vi "Begin.vi"(8 "error in":errorcluster) -> (0 "error out":errorcluster)   [LabVIEW 2017]
doc: "Called before other user functions, this VI is expected to open initial I/O refnums, load in file data, and do all program initialization. Notice that the <B>error out</B> terminal is simply used for data flow. Wiring it to other structures or subVIs ensures that this VI runs first."
uses:
  <vilib>/Rock Robotics/SystemInterfaces/DIO/FPGA_DIOPWMChannel.ctl
  <vilib>/Rock Robotics/WPI/DriverStation/WPI_DriverStationRobotMode2.ctl
  <vilib>/Rock Robotics/WPI/Joystick/WPI_JoystickDeviceEnum.ctl
  <vilib>/Rock Robotics/WPI/SafetyOutput/WPI_SafetyOutputConfigMenu.ctl
  <vilib>/Rock Robotics/WPI/RobotDrive/WPI_RobotDriveOpen2MotorWithSPARK.vi
  Robot Global Data.vi
  <vilib>/Rock Robotics/Network Tables/NT Write String Array.vi
  <vilib>/Rock Robotics/WPI/MotorControl/WPI_MotorControlOpen SPARK.vi
  <vilib>/NI_Real-Time Target Support.lvlib
panel:
  out "Led State":bool
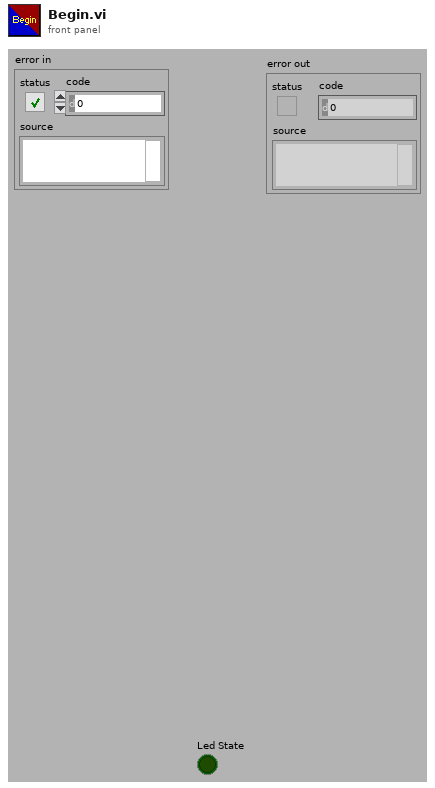
[diagram p1: front panel]
types:
  T1 = typedef "FPGA_DIOPWMChannel.ctl" = enum8{"PWM 0", "PWM 1", "PWM 2", "PWM 3", "PWM 4", "PWM 5", "PWM 6", "PWM 7", "PWM 8", "PWM 9", "PWM MXP 0", "PWM MXP 1", "PWM MXP 2", "PWM MXP 3", "PWM MXP 4", "PWM MXP 5", "PWM MXP 6", "PWM MXP 7", "PWM MXP 8", "PWM MXP 9", "Invalid"}
  T2 = typedef "WPI_SafetyOutputConfigMenu.ctl" = enum16{"Enable", "Disable"}
  T3 = typedef "WPI_JoystickDeviceEnum.ctl" = enum16{"USB 0", "USB 1", "USB 2", "USB 3", "USB 4", "USB 5"}
  T4 = typedef "WPI_DriverStationRobotMode2.ctl" = enum16{"Autonomous Disabled", "Autonomous Enabled", "Teleop Disabled", "Teleop Enabled", "Disconnected", "Finish", "Test Disabled", "Test Enabled", "Emergency Stopped"}
  T5 = typedef "WPI_JoystickDevRef.ctl" = cluster{"Device":T3}
  T6 = typedef "WPI_MotorControlDeviceRef.ctl" = cluster{"DeviceStatus":errorcluster, "Type":T7, "PWM":cluster{"PWM Channel":T1, "DeadBand":T8}, "CAN":cluster{"Device Number":u8, "SetOutput VI Ref":variant, "GetOutput VI Ref":variant, "Enable VI Ref":variant, "Disable VI Ref":variant, "Data":variant}, "Invert":bool, "DIO PWM":cluster{"PWM \"Enable\" Channel":T1, "DIOChannel":T9, "PWM Rate":dbl}}
  T7 = typedef "WPI_MotorControlType.ctl" = enum16{"PWM", "CAN", "DIO PWM"}
  T8 = typedef "WPI_PWMDeadband.ctl" = cluster{"Name":string, "maxPositivePwm":i32, "minPositivePwm":i32, "centerPwm":i32, "maxNegativePwm":i32, "minNegativePwm":i32, "angularRange":u16}
  T9 = typedef "FPGA_DIOChannel.ctl" = enum8{"DIO 0", "DIO 1", "DIO 2", "DIO 3", "DIO 4", "DIO 5", "DIO 6", "DIO 7", "DIO 8", "DIO 9", "DIO MXP 0", "DIO MXP 1", "DIO MXP 2", "DIO MXP 3", "DIO MXP 4", "DIO MXP 5", "DIO MXP 6", "DIO MXP 7", "DIO MXP 8", "DIO MXP 9", "DIO MXP 10", "DIO MXP 11", "DIO MXP 12", "DIO MXP 13", "DIO MXP 14", "DIO MXP 15", "SPI Port CS1", "SPI Port CS2", "SPI Port CS3", "SPI Port MISO", "SPI Port MOSI", "Invalid"}
  T10 = typedef "WPI_RobotDriveDevRef.ctl" = cluster{"DevStatus":errorcluster, "Motors[]":T6[], "Square Inputs":bool, "Max Output":dbl}
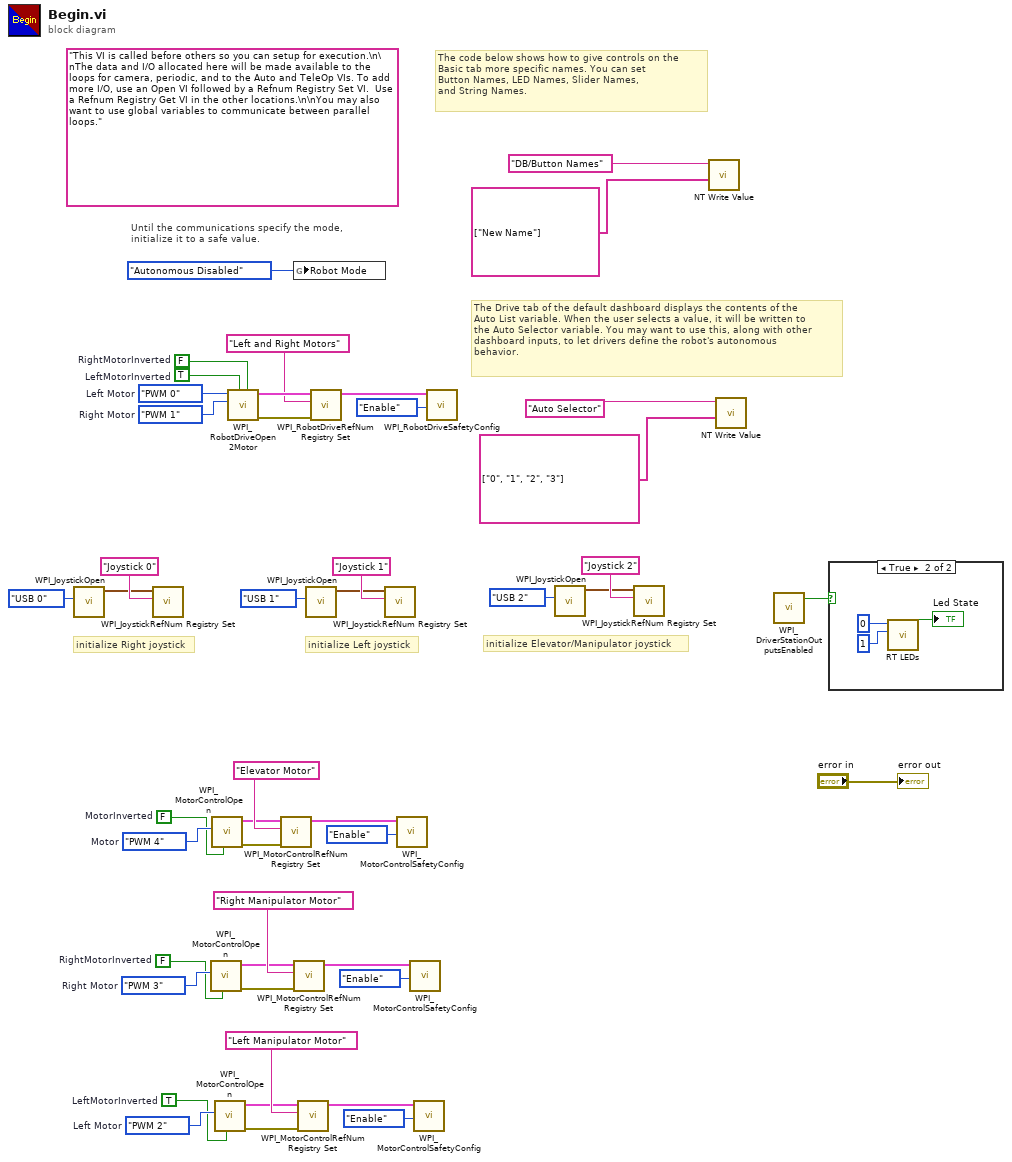
[diagram p0: block diagram]
diagram:
  w5 = FPGA_DIOPWMChannel."PWM 4"  # Motor
  w4 = FALSE  # MotorInverted
  w13 = FPGA_DIOPWMChannel."PWM 2"  # Left Motor
  w6 = TRUE  # LeftMotorInverted
  w24 = FPGA_DIOPWMChannel."PWM 3"  # Right Motor
  w7 = FALSE  # RightMotorInverted
  (unwired) "This VI is called before others so you can setup for execution.\n\nThe data and I/O allocated here will be made available to the loops for camera, periodic, and to the Auto and TeleOp VIs. To add more I/O, use an Open VI followed by a Refnum Registry Set VI.  Use a Refnum Registry Get VI in the other locations.\n\nYou may also want to use global variables to communicate between parallel loops."
  w40 = FPGA_DIOPWMChannel."PWM 1"  # Right Motor
  w41 = FPGA_DIOPWMChannel."PWM 0"  # Left Motor
  w45 = TRUE  # LeftMotorInverted
  w46 = FALSE  # RightMotorInverted
  # "initialize Elevator/Manipulator joystick"
  # "initialize Right joystick"
  # "The Drive tab of the default dashboard displays the contents of the\nAuto List variable. When the user selects a value, it will be written to\nthe Auto Selector variable. You may want to use this, along with other\ndashboard inputs, to let drivers define the robot's autonomous\nbehavior."
  # "The code below shows how to give controls on the\nBasic tab more specific names. You can set\nButton Names, LED Names, Slider Names,\nand String Names."
  # "initialize Left joystick"
  # "Until the communications specify the mode,\ninitialize it to a safe value."
  n1 = call <vilib>:"WPI_JoystickOpen.vi"("JoystickDevice"=WPI_JoystickDeviceEnum."USB 0") -> ("JoystickDevRef"=w21:T5)  [unwired: 10 in]
  n2 = call <vilib>:"WPI_JoystickRefNum Registry Set.vi"("refnum name"="Joystick 0", "JoystickDevRef"=w21) -> ()  [unwired: 8 in, 2 out]
  n3 = call-poly <vilib>:"WPI_MotorControlOpen.vi"("Invert"=w7, "PWM Channel"=w24) -> ("error out"=w25:errorcluster, "MotorControlDeviceRef"=w9:T6)  [unwired: 8 in]
  n4 = call-poly <vilib>:"WPI_MotorControlOpen.vi"("Invert"=w4, "PWM Channel"=w5) -> ("error out"=w3:errorcluster, "MotorControlDeviceRef"=w1:T6)  [unwired: 8 in]
  n5 = call-poly <vilib>:"WPI_MotorControlOpen.vi"("Invert"=w6, "PWM Channel"=w13) -> ("error out"=w14:errorcluster, "MotorControlDeviceRef"=w10:T6)  [unwired: 8 in]
  n6 = call-poly <vilib>:"WPI_RobotDriveOpen2Motor.vi"("Right Motor Inverted"=w46, "Left Motor Inverted"=w45, "Right Motor"=w40, "Left Motor"=w41) -> ("error out"=w42:errorcluster, "RobotDriveDevRef"=w44:T10)  [unwired: 6 in]
  n7 = call <vilib>:"WPI_MotorControlRefNum Registry Set.vi"("error in (no error)"=w3, "refnum name"="Elevator Motor", "MotorControlDevRef"=w1) -> ("MotorControlDevRef"=w16:T6)  [unwired: 7 in, 1 out]
  n8 = global write "Robot Global Data.vi" "Robot Mode"(WPI_DriverStationRobotMode2."Autonomous Disabled" ("Robot Mode")) -> ()
  n9 = call <vilib>:"WPI_MotorControlRefNum Registry Set.vi"("error in (no error)"=w25, "refnum name"="Right Manipulator Motor", "MotorControlDevRef"=w9) -> ("MotorControlDevRef"=w8:T6)  [unwired: 7 in, 1 out]
  n10 = call <vilib>:"WPI_MotorControlRefNum Registry Set.vi"("error in (no error)"=w14, "refnum name"="Left Manipulator Motor", "MotorControlDevRef"=w10) -> ("MotorControlDevRef"=w11:T6)  [unwired: 7 in, 1 out]
  n11 = call <vilib>:"WPI_JoystickOpen.vi"("JoystickDevice"=WPI_JoystickDeviceEnum."USB 1") -> ("JoystickDevRef"=w35:T5)  [unwired: 10 in]
  n12 = call <vilib>:"WPI_RobotDriveRefNum Registry Set.vi"("error in (no error)"=w42, "refnum name"="Left and Right Motors", "RobotDriveDevRef"=w44) -> ("RobotDriveDevRef"=w39:T10)  [unwired: 1 in, 7 out]
  n13 = call <vilib>:"WPI_JoystickRefNum Registry Set.vi"("refnum name"="Joystick 1", "JoystickDevRef"=w35) -> ()  [unwired: 8 in, 2 out]
  n14 = call <vilib>:"WPI_MotorControlSafetyConfig.vi"("mode"=WPI_SafetyOutputConfigMenu."Enable", "MotorControlDevRef"=w16) -> ()  [unwired: 8 in, 2 out]
  n15 = call <vilib>:"WPI_MotorControlSafetyConfig.vi"("mode"=WPI_SafetyOutputConfigMenu."Enable", "MotorControlDevRef"=w8) -> ()  [unwired: 8 in, 2 out]
  n16 = call <vilib>:"WPI_MotorControlSafetyConfig.vi"("mode"=WPI_SafetyOutputConfigMenu."Enable", "MotorControlDevRef"=w11) -> ()  [unwired: 8 in, 2 out]
  n17 = call <vilib>:"WPI_RobotDriveSafetyConfig.vi"("mode"=WPI_SafetyOutputConfigMenu."Enable", "RobotDriveDevRef"=w39) -> ()  [unwired: 8 in, 2 out]
  n18 = call <vilib>:"WPI_JoystickOpen.vi"("JoystickDevice"=WPI_JoystickDeviceEnum."USB 2") -> ("JoystickDevRef"=w18:T5)  [unwired: 10 in]
  n19 = call <vilib>:"WPI_JoystickRefNum Registry Set.vi"("refnum name"="Joystick 2", "JoystickDevRef"=w18) -> ()  [unwired: 8 in, 2 out]
  n20 = call-poly <vilib>:"NT Write Value.vi"("String Array"=string[] ["New Name"], "Name"="DB/Button Names") -> ()  [unwired: 9 in, 1 out]
  n21 = call-poly <vilib>:"NT Write Value.vi"("String Array"=string[] ["0", "1", "2", "3"], "Name"="Auto Selector") -> ()  [unwired: 9 in, 1 out]
  n22 = call <vilib>:"WPI_DriverStationOutputsEnabled.vi"() -> ("OutputsEnabled?"=w28:bool)  [unwired: 10 in, 1 out]
  n23 = case shown="True" w28 {
    frame False {
    }
    frame True {
      n24 = call <vilib>:"RT LEDs.vi"("State"=1, "LED Num"=0) -> ("Led State"=→"Led State":bool)  [unwired: 4 in, 1 out]
    }
  }
  "error out" <- "error in"
